vi "Main.vi"() -> ()   [LabVIEW 2014, in "SLL Add Copyright.lvlib"]
uses:
  SLL Add Copyright.lvlib
  Typedefs/Select Type.ctl
panel:
  out "Progress":i32(slide) scale=0.0..5.0
  in  "Type":T1={"vi"=TRUE, "ctl"=TRUE, "lvlib"=TRUE, "lvclass"=TRUE, "lvproj"=TRUE} caption="Select File Type to Add Copyright"
  in  "Folder":path
  in  "Copyright Text":string="© Company Name"
  out "error out":errorcluster
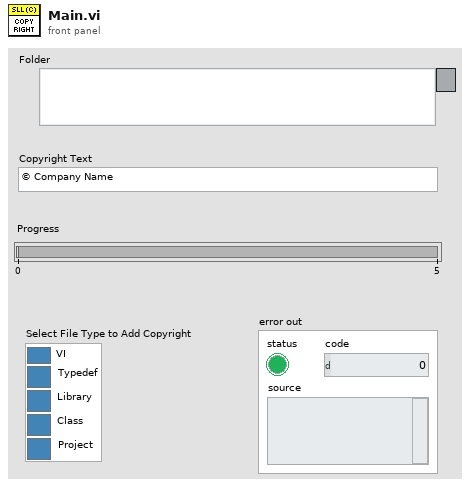
[diagram p1: front panel]
types:
  T1 = typedef "SLL Add Copyright.lvlib/Select Type.ctl" = cluster{"vi":bool, "ctl":bool, "lvlib":bool, "lvclass":bool, "lvproj":bool}
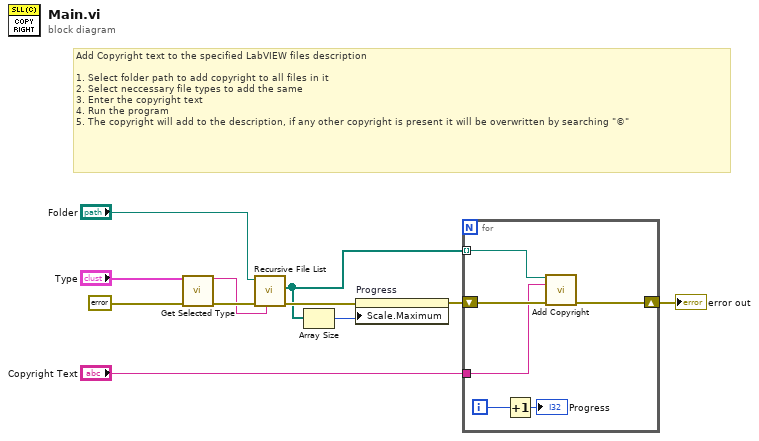
[diagram p0: block diagram]
diagram:
  # "Add Copyright text to the specified LabVIEW files description\n\n1. Select folder path to add copyright to all files in it\n2. Select neccessary file types to add the same\n3. Enter the copyright text\n4. Run the program\n5. The copyright will add to the description, if any other copyright is present it will be overwritten by searching \"©\""
  n1 = call "Get Selected Type.vi"("Select Type"="Type", "error in (no error)"=errorcluster {"status"=FALSE, "code"=0, "source"=""}) -> ("Selected Type Pattern"=w4:string, "error out"=w7:errorcluster)  [unwired: 12 in]
  n2 = call <vilib>:"Recursive File List.vi"("pattern"=w4, "error in (no error)"=w7, "Folder Path"="Folder") -> ("error out"=w6:errorcluster, "All Files in Dir"=w3:path[])  [unwired: 4 in, 3 out]
  n3 = Array Size(array=w3) -> (size(s)=w2:i32)
  n4 = property on="Progress" class="Slide (strict)"(error in=w6, "Scale.Maximum"=w2) -> (error out=w8:errorcluster)  [unwired: 1 in, 1 out]
  n5 = for {
    shift-right: [w15] -> w11
    shift-left: w8 -> [w16]
    tunnel: w3 -> [w17] mode=indexing
    tunnel: "Copyright Text" -> [w12]
    i -> [w14]
    n6 = Increment(x=w14) -> (x+1=→"Progress":i32)
    n7 = call "Add Copyright.vi"("File Path"=w17, "Copyright Text"=w12, "error in (no error)"=w16) -> ("error out"=w15:errorcluster)  [unwired: 12 in]
  }
  "error out" <- w11
